vi "Test - 1.vi"() -> ()   [LabVIEW 2013]
uses:
  Item/Item.lvclass
  Generic/Generic.lvclass
panel:
  out "Modified":bool
  out "ClassName":string
  out "ClassID":u32
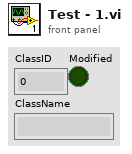
[diagram p1: front panel]
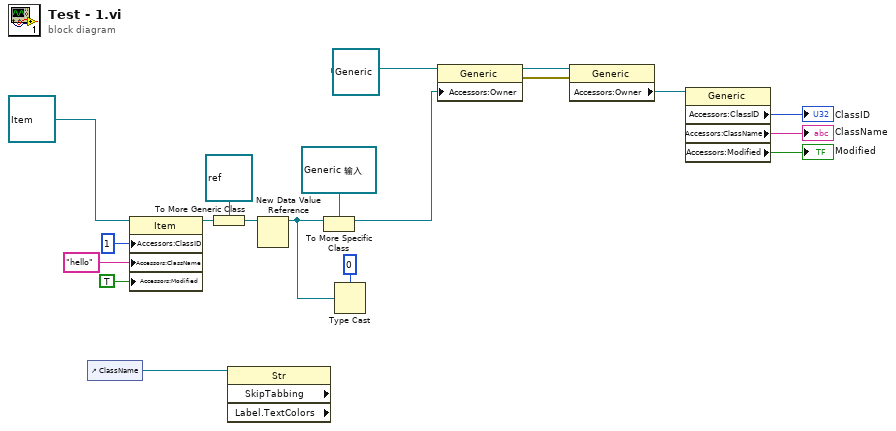
[diagram p0: block diagram]
diagram:
  n1 = control-ref of="ClassName"() -> (w5:refnum<vi>)
  n2 = property class="Item"(reference=refnum<class "Item.lvclass"> refnum ("Framework.lvlib:Item"), "Accessors:ClassID"=u32 1 ("ClassID"), "Accessors:ClassName"="hello" ("ClassName"), "Accessors:Modified"=TRUE ("Modified")) -> (reference out=w15:refnum<class "Item.lvclass">)  [unwired: 1 in, 1 out]
  n3 = To More Generic Class(target class=refnum<class> refnum ("LabVIEW Object"), reference=w15) -> (generic class reference=w13:refnum<class>)
  n4 = property class="Str" props=["SkipTabbing", "Label", "TextColors"](reference=w5) -> ()  [unwired: 1 in, 4 out]
  n5 = New Data Value Reference(data value=w13) -> (data value reference=w8:refnum<data-value>)  [unwired: 1 in, 1 out]
  n6 = To More Specific Class(target class=refnum<data-value> refnum ("Owner"), reference=w8) -> (specific class reference=w1:refnum<data-value>)  [unwired: 1 in, 1 out]
  n7 = Type Cast(type=u64 0, x=w8) -> ()  [unwired: 1 out]
  n8 = property class="Generic"(reference=refnum<class "Generic.lvclass"> refnum ("Framework.lvlib:Generic"), "Accessors:Owner"=w1) -> (reference out=w19:refnum<class "Generic.lvclass">, error out=w18:errorcluster)  [unwired: 1 in]
  n9 = property class="Generic"(reference=w19, error in=w18) -> ("Accessors:Owner"=w9:refnum<data-value>)  [unwired: 2 out]
  n10 = property class="Generic"(reference=w9) -> ("Accessors:ClassID"=→"ClassID":u32, "Accessors:ClassName"=→"ClassName":string, "Accessors:Modified"=→"Modified":bool)  [unwired: 1 in, 2 out]
